vi "set_package_attribute_string.vi"() -> ()   [LabVIEW 2020]
uses:
  dragon_toml_64.dll
panel:
  out "set":bool
  in  "attribute_name":string="version"
  in  "attribute_value":string="2023.3.0"
  in  "file_path":path=path "C:/Projects/labview-project-load-tools/rust_src/toml_edit_dll/lv_src/test.toml"
  out "error out":errorcluster
  in  "package":string="ni-daqmx"
  in  "package_manager":string="nipm"
  in  "error in (no error)":errorcluster
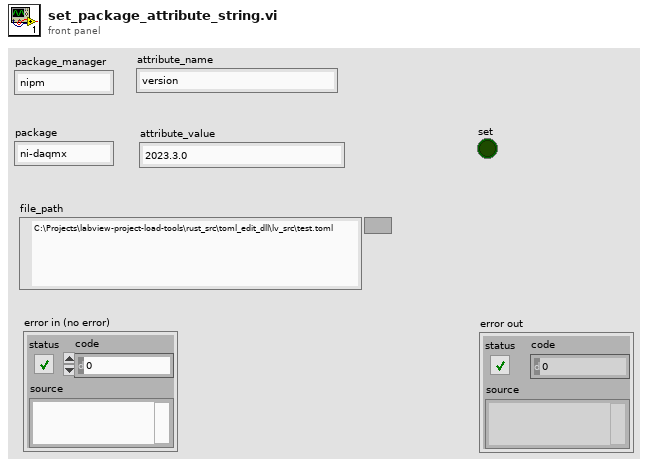
[diagram p1: front panel]
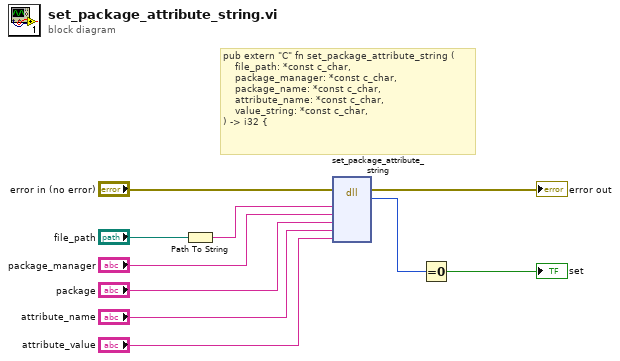
[diagram p0: block diagram]
diagram:
  # "pub extern \"C\" fn set_package_attribute_string (\n    file_path: *const c_char,\n    package_manager: *const c_char,\n    package_name: *const c_char,\n    attribute_name: *const c_char,\n    value_string: *const c_char,\n) -> i32 {"
  n1 = Path To String(path="file_path") -> (string=w6:string)
  n2 = dll-call lib="C:/Projects/toml-edit-labview/lv_src/dragon_toml_*.dll" fn="set_package_attribute_string"(error in="error in (no error)", "file_path"=w6, "package_manager"="package_manager", "package_name"="package", "attribute_name"="attribute_name", "attribute_value"="attribute_value") -> (error out=→"error out":errorcluster, "result"=w1:i32)  [unwired: 7 in, 1 out]
  n3 = Equal To 0?(x=w1) -> (x = 0?=→"set":bool)
